vi "Append String.vi"(8 "error in":errorcluster, 11 "String to Append":string) -> (0 "error out":errorcluster, 3 "String Out":string)   [LabVIEW 2014]
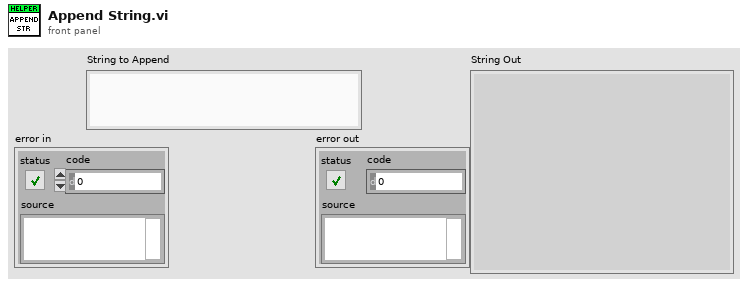
[diagram p1: front panel]
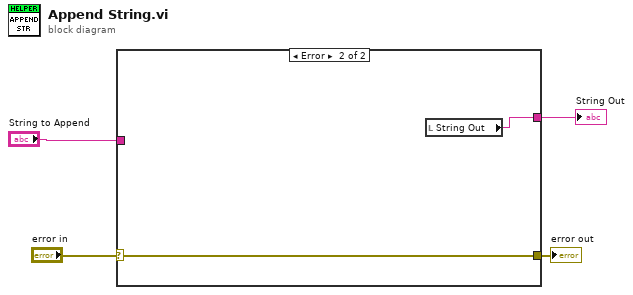
[diagram p0: block diagram]
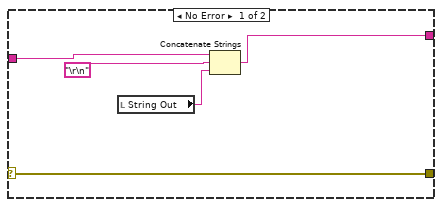
[diagram p2: hidden frame]
diagram:
  n1 = case shown="Error" "error in" {
    selector: "error in" -> [w9 w11]
    tunnel: [w9 w11] -> w3
    tunnel: "String to Append" -> [w6 _]
    tunnel: [w5 w10] -> w1
    frame No Error {
      n2 = local read "String Out"() -> (w8:string)
      n3 = Concatenate Strings(w6, "\r\n", w8) -> (w5:string)
    }
    frame Error {
      n4 = local read "String Out"() -> (w10:string)
    }
  }
  "error out" <- w3
  "String Out" <- w1
